vi "Comms Client.vi"(6 "Read response":bool, 7 "Keep alive":dbl=100.0 format="%#_6ps", 8 "Error In":errorcluster, 9 "Message":string, 10 "Service name":string="LabActor Comms", 11 "Address":string="127.0.0.1") -> (0 "Error Out":errorcluster, 1 "Valid response":bool, 2 "Response":string, 3 "connection ID out":refnum<k5>)   [LabVIEW 2016]
doc: "TCP communication client with running LabActor application. Make sure LabActor.cfg includes \"TCP Communications\""
panel:
  # "Supported messages\n\nCommands:\nSET START\nSET STOP\n\nQueries:\nGET Monitor State\nGET Spectrum Recorder\nGET Line Detector"
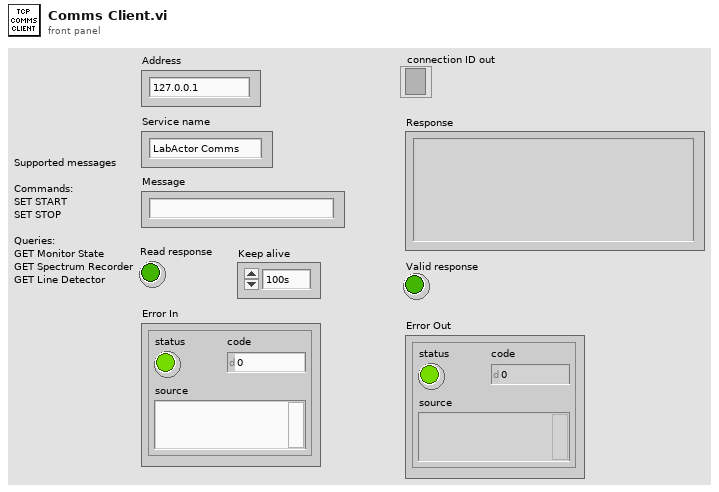
[diagram p1: front panel]
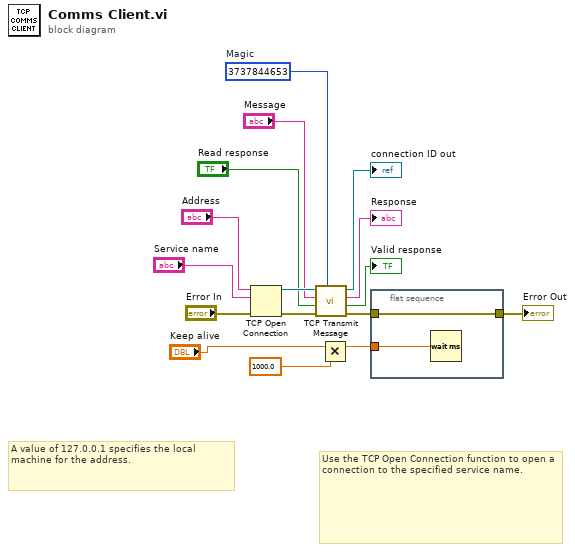
[diagram p0: block diagram]
diagram:
  w13 = u32 3737844653  # Magic
  # "Use the TCP Open Connection function to open a connection to the specified service name."
  # "A value of 127.0.0.1 specifies the local machine for the address."
  n1 = TCP Open Connection(address="Address", remote port or service name="Service name", error in (no error)="Error In") -> (connection ID=w14:refnum<k5>, error out=w9:errorcluster)  [unwired: 2 in]
  n2 = call "TCP Transmit Message.vi"("Magic"=w13, "Error In"=w9, "Wait for response"="Read response", "Message"="Message", "connection ID"=w14) -> ("Error Out"=w5:errorcluster, "Valid response"=→"Valid response":bool, "Response"=→"Response":string, "connection ID out"=→"connection ID out":refnum<k5>)  [unwired: 3 in]
  n3 = Multiply(x="Keep alive", y=1000.0) -> (x*y=w2:dbl)
  n4 = flat-sequence {
    tunnel: w5 -> [w18]
    tunnel: [w18] -> w4
    tunnel: w2 -> [w17]
    frame #0 {
      n5 = Wait (ms)(milliseconds to wait=w17) -> ()  [unwired: 1 out]
    }
  }
  "Error Out" <- w4
